vi "us test.vi"() -> ()   [LabVIEW 2019]
uses:
  <vilib>/Platform/TimedLoop/XDataNode/timing_clust.ctl
  <vilib>/Platform/TimedLoop/XDataNode/nitl_modes.ctl
  <vilib>/Platform/TimedLoop/XDataNode/wakeup.ctl
  FPGA_subVIs/low level/us sensor/US sensor.lvclass
  <vilib>/platform/TimedLoop/XDataNode/XDataNode.xnode
  <vilib>/Platform/TimedLoop/XDataNode/XDNodeRunTimeDep.lvlib
panel:
  out "Waveform Chart":dbl(graph)
  in  "Stop":bool
  out "DC estimate (V)":dbl format="%0.2f"
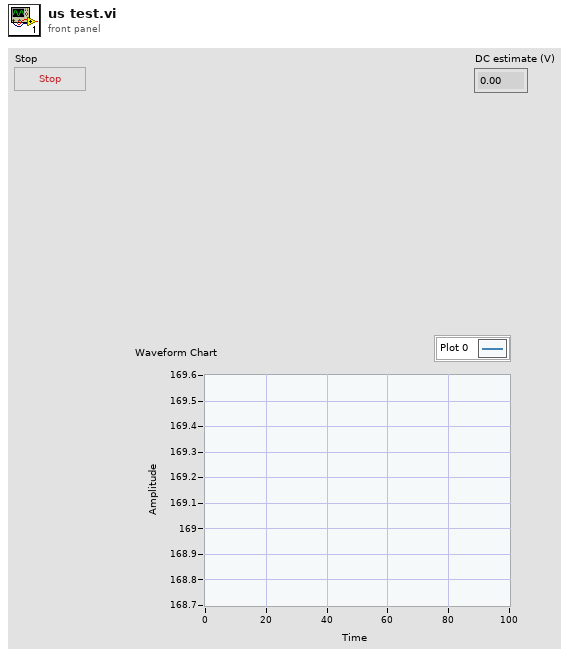
[diagram p1: front panel]
types:
  T1 = typedef "XDNodeRunTimeDep.lvlib/timing_clust.ctl" = cluster{"Expected End [f-1]":u64, "Actual End [f-1]":u64, "Finished Late? [f-1]":bool, "Expected End [i-1]":u64, "Actual End [i-1]":u64, "Finished Late? [i-1]":bool, "Expected Start [i]":u64, "Actual Start [i]":u64, "Expected Start [f]":u64, "Actual Start [f]":u64, "Source Name":string, "Structure Name":string, "Period":i64, "Deadline":i64, "Offset":i64, "Start":i64, "Priority":i32, "Timeout":i32, "Mode":T2, "Wakeup Reason":T3, "Error":errorcluster, "Source Type":string, "Secondary Source Type":string, "Global End Time":u64, "Global Start Time":u64, "Frame Duration":u64, "Iteration Duration":u64, "Assigned CPU":i32, "I/O Scan Engine Mode":u32}
  T2 = typedef "XDNodeRunTimeDep.lvlib/nitl_modes.ctl" = enum32{"No Change", "Process missed periods, maintain original phase", "Discard missed periods, maintain original phase", "Process missed periods, ignore original phase", "Discard missed periods, ignore original phase"}
  T3 = typedef "XDNodeRunTimeDep.lvlib/wakeup.ctl" = enum32{"Normal", "Aborted", "Asynchronous wakeup", "Timing source error", "Timed loop error", "Timeout"}
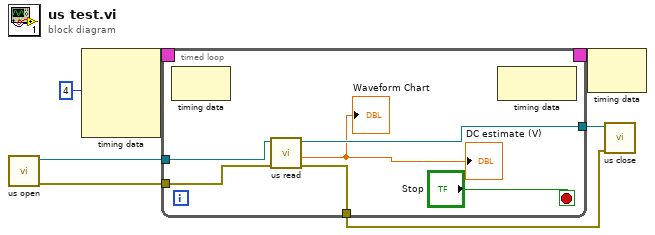
[diagram p0: block diagram]
diagram:
  n1 = call "us open.vi"() -> ("error out"=w4:errorcluster, "output cluster"=w5:refnum<class "US sensor.lvclass">)  [unwired: 10 in]
  n2 = node-c288(i64 4 ("Period")) -> (w7:T1)  [unwired: 3 in]
  n3 = timed-loop {
    timing: w7 -> [_]
    timing-out: [_] -> w6
    tunnel: w5 -> [w13]
    tunnel: w4 -> [w12]
    tunnel: [w10] -> w2
    tunnel: [w9] -> w1
    stop <- "Stop" stop-if-true
    n4 = node-c288() -> ()  [unwired: 1 in, 1 out]
    n5 = call "us read.vi"("Error In"=w12, "my FPGA lib.lvlib:US sensor.lvclass"=w13) -> ("error out"=w10:errorcluster, "DC estimate (V)"=→"DC estimate (V)" →"Waveform Chart":dbl, "my FPGA lib.lvlib:US sensor.lvclass 2"=w9:refnum<class "US sensor.lvclass">)  [unwired: 5 in, 2 out]
    n6 = node-c288() -> ()  [unwired: 1 in, 1 out]
  }
  n7 = node-c288(w6) -> ()  [unwired: 1 out]
  n8 = call "us close.vi"("Error In"=w2, "my FPGA lib.lvlib:US sensor.lvclass"=w1) -> ()  [unwired: 9 in, 1 out]
